vi "CytecControl.vi"(3 "SwitchMatrix":bool[][](array[boolean]), 4 "VISA resource name":refnum<visa-resource-name>="Cytec_Switch") -> ()   [LabVIEW 2021]
panel:
  in  "DisconnectAll":bool
  in  "error in (no error)":errorcluster
  in  "GroundAll":bool
  in  "Set":bool
  in  "Read":bool
  out "error out":errorcluster
  in  "Quit":bool
  in  "SamplePins":string[](array[string])=["23", "18", "15", "14", "13", "12", "24", "1", "10", "11"]
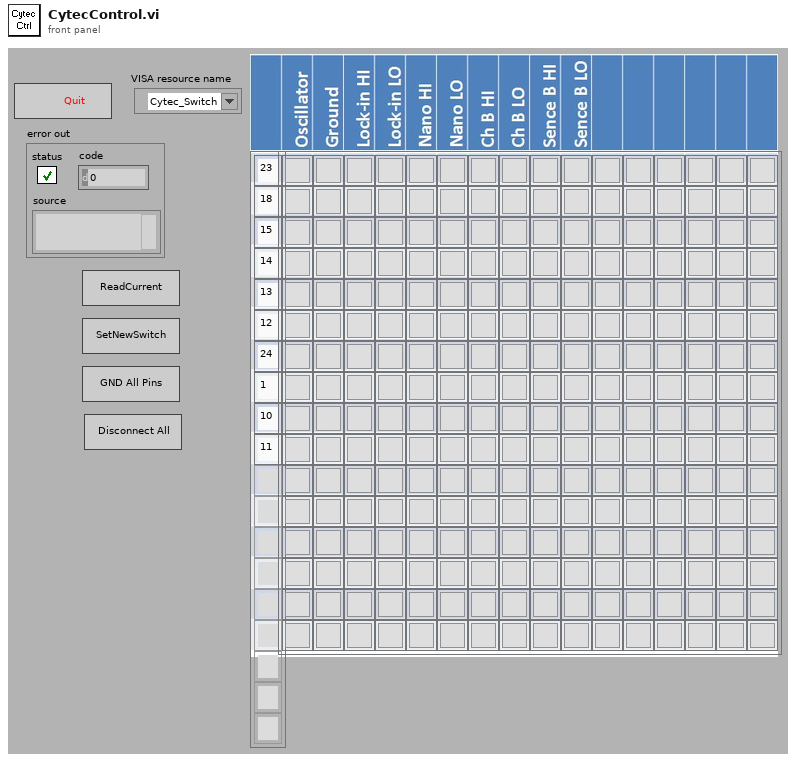
[diagram p1: front panel]
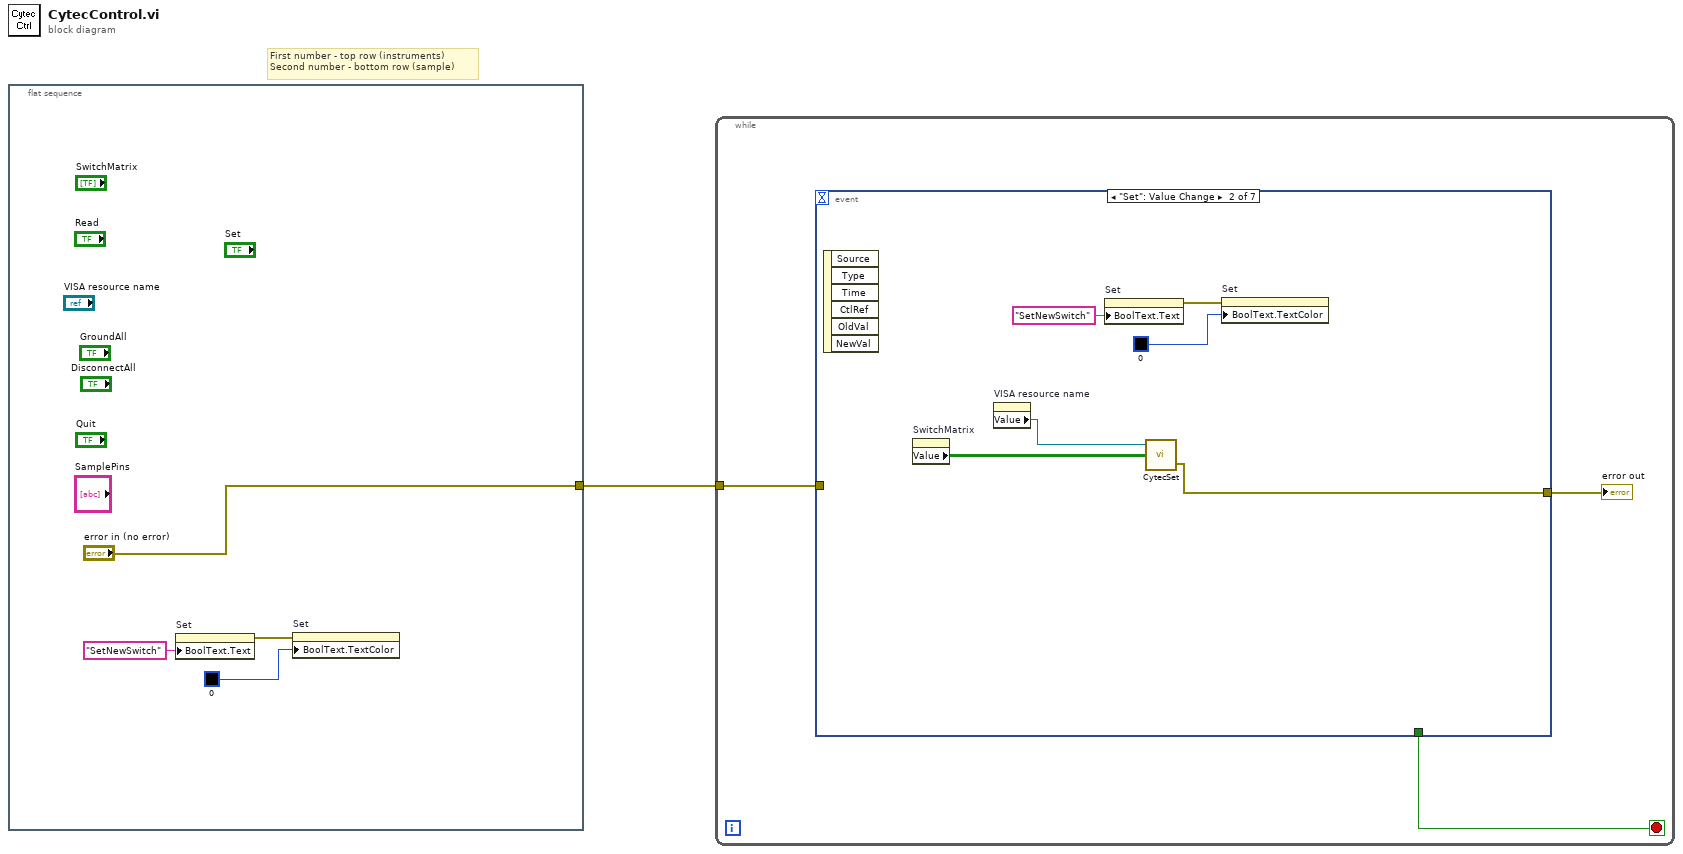
[diagram p0: block diagram]
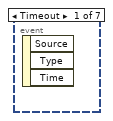
[diagram p2: hidden frame]
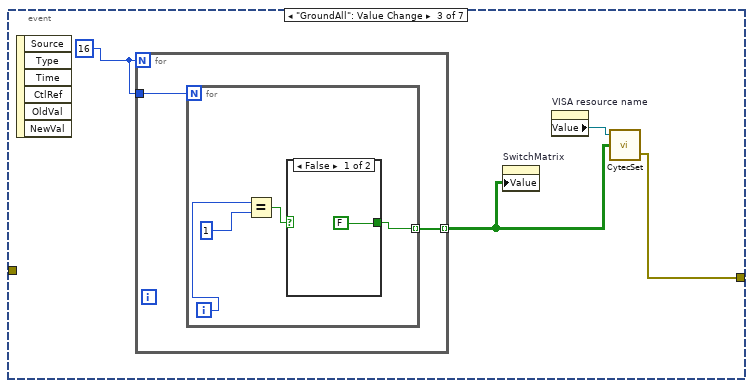
[diagram p3: hidden frame]
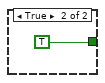
[diagram p4: hidden frame]
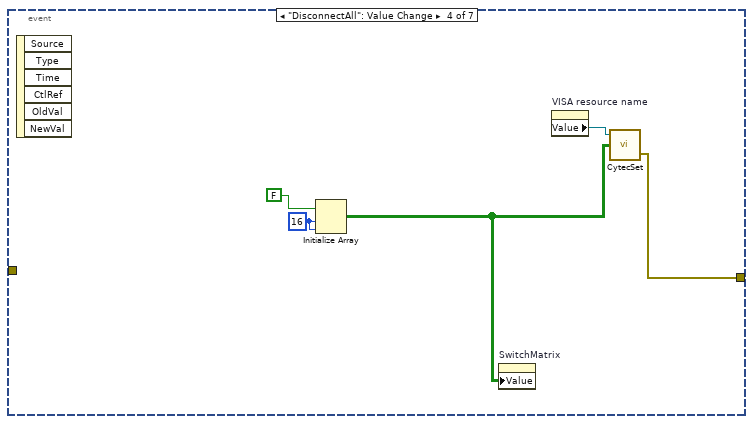
[diagram p5: hidden frame]
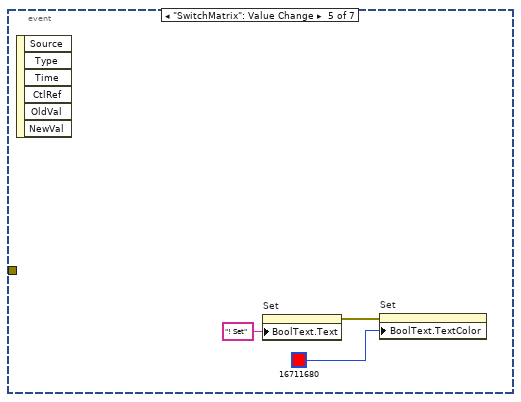
[diagram p6: hidden frame]
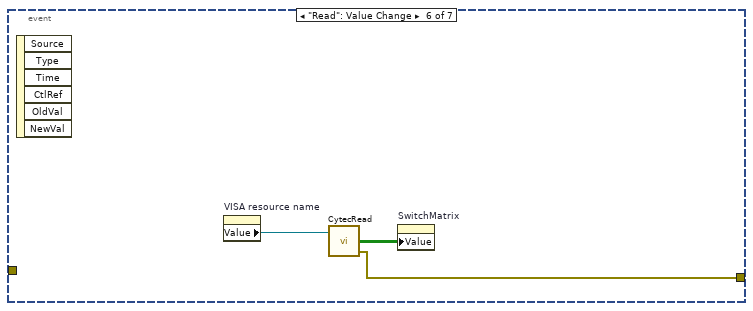
[diagram p7: hidden frame]
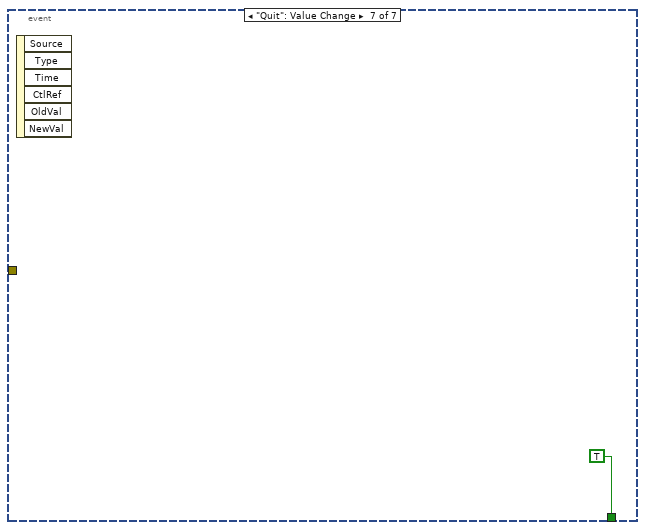
[diagram p8: hidden frame]
diagram:
  # "First number - top row (instruments)\nSecond number - bottom row (sample)"
  n1 = flat-sequence {
    tunnel: ["error in (no error)"] -> w1
    frame #0 {
      n2 = property on="Set" class="Bool"("BoolText.Text"="SetNewSwitch" ("Boolean Text.Text")) -> (error out=w4:errorcluster)  [unwired: 2 in, 1 out]
      n3 = property on="Set" class="Bool"(error in=w4, "BoolText.TextColor"=u32 0 ("Boolean Text.Text Colors:Text Color")) -> ()  [unwired: 1 in, 2 out]
    }
  }
  n4 = while {
    tunnel: w1 -> [w6]
    stop <- w7 stop-if-true
    n5 = event shown="[1] \"Set\": Value Change" {
      selector: _ -> [_ _ _ _ _ _ _]
      dyn-events: _ -> [_ _ _ _ _ _ _]
      timeout: _ -> [_ _ _ _ _ _ _]
      tunnel: [_ w12 w15 w30 _ w35 _] -> w8
      tunnel: [_ _ _ _ _ _ TRUE] -> w7
      tunnel: w6 -> [_ _ _ _ _ _ _]
      event Timeout {
        n6 = event-data() -> ()  [unwired: 1 in, 3 out]
      }
      event "Set": Value Change {
        n7 = event-data() -> ()  [unwired: 1 in, 6 out]
        n8 = property on="SwitchMatrix" class="Arr (strict)"() -> ("Value"=w14:bool[][])  [unwired: 2 in, 2 out]
        n9 = property on="VISA resource name" class="VISAName"() -> ("Value"=w13:refnum<visa-resource-name>)  [unwired: 2 in, 2 out]
        n10 = property on="Set" class="Bool"("BoolText.Text"="SetNewSwitch" ("Boolean Text.Text")) -> (error out=w9:errorcluster)  [unwired: 2 in, 1 out]
        n11 = call "CytecSet.vi"("SwitchMatrix"=w14, "VISA resource name"=w13) -> ("error out"=w12:errorcluster)  [unwired: 1 in, 1 out]
        n12 = property on="Set" class="Bool"(error in=w9, "BoolText.TextColor"=u32 0 ("Boolean Text.Text Colors:Text Color")) -> ()  [unwired: 1 in, 2 out]
      }
      event "GroundAll": Value Change {
        w18 = 16
        n13 = event-data() -> ()  [unwired: 1 in, 6 out]
        n14 = for {
          N: w18 -> [_]
          tunnel: w18 -> [w20]
          tunnel: [w19] -> w16 mode=indexing
          n15 = for {
            N: w20 -> [_]
            tunnel: [w22] -> w19 mode=indexing
            i -> [w21]
            n16 = Equal?(x=w21, y=1) -> (x = y?=w23:bool)
            n17 = case shown="False" w23 {
              tunnel: [FALSE TRUE] -> w22
              frame False {
              }
              frame True {
              }
            }
          }
        }
        n18 = property on="SwitchMatrix" class="Arr (strict)"("Value"=w16) -> ()  [unwired: 2 in, 2 out]
        n19 = property on="VISA resource name" class="VISAName"() -> ("Value"=w17:refnum<visa-resource-name>)  [unwired: 2 in, 2 out]
        n20 = call "CytecSet.vi"("SwitchMatrix"=w16, "VISA resource name"=w17) -> ("error out"=w15:errorcluster)  [unwired: 1 in, 1 out]
      }
      event "DisconnectAll": Value Change {
        w28 = 16 ("dimension size")
        n21 = event-data() -> ()  [unwired: 1 in, 6 out]
        n22 = Initialize Array(FALSE, w28, w28) -> (w27:bool[][])
        n23 = property on="SwitchMatrix" class="Arr (strict)"("Value"=w27) -> ()  [unwired: 2 in, 2 out]
        n24 = property on="VISA resource name" class="VISAName"() -> ("Value"=w31:refnum<visa-resource-name>)  [unwired: 2 in, 2 out]
        n25 = call "CytecSet.vi"("SwitchMatrix"=w27, "VISA resource name"=w31) -> ("error out"=w30:errorcluster)  [unwired: 1 in, 1 out]
      }
      event "SwitchMatrix": Value Change {
        n26 = event-data() -> ()  [unwired: 1 in, 6 out]
        n27 = property on="Set" class="Bool"("BoolText.Text"="! Set" ("Boolean Text.Text")) -> (error out=w32:errorcluster)  [unwired: 2 in, 1 out]
        n28 = property on="Set" class="Bool"(error in=w32, "BoolText.TextColor"=u32 16711680 ("Boolean Text.Text Colors:Text Color")) -> ()  [unwired: 1 in, 2 out]
      }
      event "Read": Value Change {
        n29 = event-data() -> ()  [unwired: 1 in, 6 out]
        n30 = property on="VISA resource name" class="VISAName"() -> ("Value"=w37:refnum<visa-resource-name>)  [unwired: 2 in, 2 out]
        n31 = call "CytecRead.vi"("VISA resource name"=w37) -> ("error out"=w35:errorcluster, "SwitchMatrix"=w36:bool[][])  [unwired: 2 in, 1 out]
        n32 = property on="SwitchMatrix" class="Arr (strict)"("Value"=w36) -> ()  [unwired: 2 in, 2 out]
      }
      event "Quit": Value Change {
        n33 = event-data() -> ()  [unwired: 1 in, 6 out]
      }
    }
    "error out" <- w8
  }
